vi "Publisher_SM.vi"() -> ()   [LabVIEW 2015]
uses:
  Data.ctl
  <vilib>/daq.io/MQTT LabVIEW Client/Controls/QoS.ctl
  <vilib>/daq.io/MQTT LabVIEW Client/Controls/Retain_Flag.ctl
  <vilib>/daq.io/MQTT LabVIEW Client/Controls/DUP_Flag.ctl
  <vilib>/daq.io/MQTT LabVIEW Client/Controls/Connection_Return_Codes.ctl
  Battery Controller.ctl
  States.ctl
  <vilib>/myRIO/Instrument Drivers/Onboard IO/DIO/typedefs/DIO Reference.ctl
  <vilib>/myRIO/Common/Instrument Driver Framework/Utilities/typedefs/myRIO Generic Hardware Reference.ctl
  <vilib>/myRIO/Common/Instrument Driver Framework/Utilities/typedefs/Hardware Version Enum.ctl
  <vilib>/myRIO/Common/Instrument Driver Framework/Utilities/typedefs/myRIO v1.0 Reference.ctl
  <vilib>/myRIO/Common/Instrument Driver Framework/Utilities/typedefs/Generic FPGA Reference.ctl
  <vilib>/myRIO/Common/Instrument Driver Framework/myRIO v1.0/DIO/typedefs/DIO Channels List.ctl
  <vilib>/myRIO/Common/Instrument Driver Framework/myRIO v1.0/DIO/typedefs/DIO Channels Enum.ctl
  <vilib>/userdefined/High Color/nirio_resource_hc.ctl
  <vilib>/myRIO/Common/Instrument Driver Framework/Utilities/vis/Is FPGA Ref Available.vi
  <vilib>/myRIO/Common/Instrument Driver Framework/myRIO v1.0/DIO/vis/myRIO v1.1 Open DIO.vi
  <vilib>/myRIO/Instrument Drivers/Onboard IO/DIO/vis/Read.vi
  <vilib>/myRIO/Instrument Drivers/Onboard IO/DIO/vis/Write.vi
  <vilib>/myRIO/Common/Instrument Driver Framework/Utilities/vis/Validate Channels.vi
  <vilib>/myRIO/Common/Instrument Driver Framework/myRIO v1.0/DIO/vis/myRIO v1.0 Reserve DIO.vi
  <vilib>/myRIO/Common/Instrument Driver Framework/myRIO v1.0/Resource Manager/vis/myRIO v1.0 Reserve Channel List.vi
  <vilib>/myRIO/Common/Instrument Driver Framework/myRIO v1.0/DIO/vis/myRIO v1.0 Build MUX Configuration DIO.vi
  <vilib>/myRIO/Common/Instrument Driver Framework/myRIO v1.0/Resource Manager/vis/myRIO v1.0 Reserve Channel.vi
  <vilib>/myRIO/Common/Instrument Driver Framework/myRIO v1.0/Resource Manager/vis/myRIO v1.0 Unreserve Channel.vi
  <vilib>/myRIO/Common/Instrument Driver Framework/myRIO v1.0/Resource Manager/vis/myRIO v1.0 Create Configuration List.vi
  <vilib>/myRIO/Common/Instrument Driver Framework/myRIO v1.0/Resource Manager/vis/myRIO v1.0 Build Mutex Name.vi
  <vilib>/Instr/_visa.llb/VISA Configure Serial Port (Instr).vi
  <vilib>/Utility/VariantDataType/GetNumericInfo.vi
  <vilib>/Utility/error.llb/Error Cluster From Error Code.vi
  <vilib>/myRIO/Common/Instrument Driver Framework/myRIO v1.0/myRIO v1.1 Open.vi
  <vilib>/myRIO/Common/Instrument Driver Framework/Utilities/vis/IO Manager.vi
  <vilib>/myRIO/Common/Instrument Driver Framework/Utilities/vis/Configuration Manager.vi
  <vilib>/myRIO/Common/Instrument Driver Framework/myRIO v1.0/Resource Manager/vis/myRIO v1.0 Configure IO.vi
  <vilib>/myRIO/Common/Instrument Driver Framework/myRIO v1.0/myRIO v1.0 Close.vi
  <vilib>/myRIO/Common/Instrument Driver Framework/myRIO v1.0/DIO/vis/myRIO v1.0 Read DIO.vi
  <vilib>/myRIO/Common/Instrument Driver Framework/myRIO v1.0/DIO/vis/myRIO v1.0 Write DIO.vi
  <vilib>/myRIO/Express VI/Onboard Devices/Button/Button Express VI.xnode
  <vilib>/myRIO/Instrument Drivers/Onboard IO/DIO/vis/myRIO DIO Open.xnode
  <vilib>/myRIO/Express VI/Onboard Devices/LED/LED Express VI.xnode
  <vilib>/daq.io/MQTT LabVIEW Client/MQTT_Functions.lvlib
  <vilib>/myRIO/Instrument Drivers/Onboard IO/DIO/DIO.lvlib
panel:
  in  "Battery Controls":T1={"Battery Serial Port"="ASRL2::INSTR", "Command to write"="RD_STAT>\r"}
  out "error out":errorcluster
  out "Session Status":string
  out "Published Data":string[][](array[string])
  in  "Stop Button":bool
  out "Connection Status":T2=enum."Connection refused: not authorized"
  in  "Connection Paramaters":T3={"VISA resource name"="ASRL1::INSTR", "myRIO AI Channel"=["C/AI0", "C/AI1"], "baud rate (9600)"=19200, "Write Command"="0R0!", "Client ID"="myRIO", "Topic"="All Weather Data", "Message ID"=10, "MQTT Broker"={"address (IP)"="52.38.228.154", "port"=1883}, "Publish Meta"={"QoS"=enum."At most once", "Retain"=FALSE, "DUP"=FALSE}, "TCP connection ID "=refnum, "Session Status"=""}
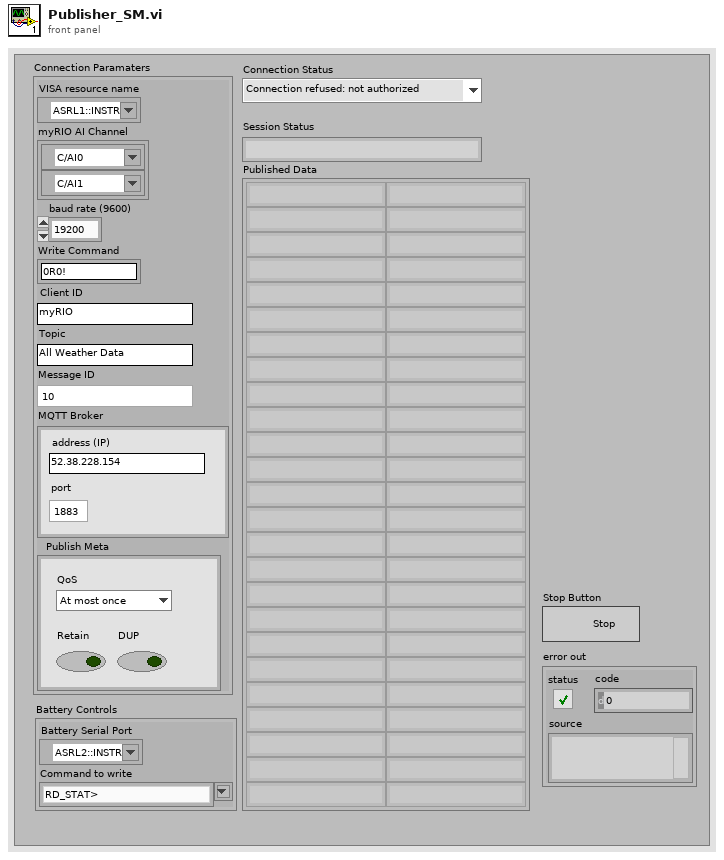
[diagram p1: front panel]
types:
  T1 = typedef "Battery Controller.ctl" = cluster{"Battery Serial Port":refnum<visa-resource-name>, "Command to write":string}
  T2 = typedef "MQTT_Functions.lvlib/Connection_Return_Codes.ctl" = enum16{"Connection accepted", "Connection refused: unacceptable protocol version", "Connection refused: identifier rejected", "Connection refused: Server unavailable", "Connection refused: bad user name or password", "Connection refused: not authorized"}
  T3 = typedef "Data.ctl" = cluster{"VISA resource name":refnum<visa-resource-name>, "myRIO AI Channel":tag[], "baud rate (9600)":u32, "Write Command":string, "Client ID":string, "Topic":string, "Message ID":u16, "MQTT Broker":cluster{"address (IP)":string, "port":u16}, "Publish Meta":cluster{"QoS":T4, "Retain":T5, "DUP":T6}, "TCP connection ID ":refnum<k5>, "Session Status":string}
  T4 = typedef "MQTT_Functions.lvlib/QoS.ctl" = enum8{"At most once", "At least once", "Exactly once", "Reserved"}
  T5 = typedef "MQTT_Functions.lvlib/Retain_Flag.ctl" = bool
  T6 = typedef "MQTT_Functions.lvlib/DUP_Flag.ctl" = bool
  T7 = typedef "States.ctl" = enum16{"Initialize", "TCP Connect", "Gather/Publish", "TCP Ping", "Exit/Disconnect"}
  T8 = typedef "DIO.lvlib/DIO Reference.ctl" = cluster{"myRIO Reference":T9, "DIO Channels List":T13}
  T9 = typedef "myRIO Generic Hardware Reference.ctl" = cluster{"myRIO Model":T10, "myRIO Hardware Reference":T11}
  T10 = typedef "Hardware Version Enum.ctl" = enum16{"Unknown", "myRIO-1900", "myRIO-1950", "roboRIO"}
  T11 = typedef "myRIO v1.0 Reference.ctl" = cluster{"Generic FPGA Reference":T12, "Allow multiple opens":bool}
  T12 = typedef "Generic FPGA Reference.ctl" = refnum<k20>
  T13 = typedef "DIO Channels List.ctl" = T14[]
  T14 = typedef "DIO Channels Enum.ctl" = enum16{"Not Connected", "C/DIO0", "C/DIO1", "C/DIO2", "C/DIO3", "C/DIO4", "C/DIO5", "C/DIO6", "C/DIO7", "A/DIO0", "A/DIO1", "A/DIO2", "A/DIO3", "A/DIO4", "A/DIO5", "A/DIO6", "A/DIO7", "A/DIO8", "A/DIO9", "A/DIO10", "A/DIO11", "A/DIO12", "A/DIO13", "A/DIO14", "A/DIO15", "B/DIO0", "B/DIO1", "B/DIO2", "B/DIO3", "B/DIO4", "B/DIO5", "B/DIO6", "B/DIO7", "B/DIO8", "B/DIO9", "B/DIO10", "B/DIO11", "B/DIO12", "B/DIO13", "B/DIO14", "B/DIO15", "LED0", "LED1", "LED2", "LED3", "Button0", "DIO/DIO0", "DIO/DIO1", "DIO/DIO2", "DIO/DIO3", "DIO/DIO4", "DIO/DIO5", "DIO/DIO6", "DIO/DIO7", "DIO/DIO8", "DIO/DIO9", "SPI/CS0", "SPI/CS1", "SPI/CS2", "SPI/CS3", "LED RADIO (Green)", "LED RADIO (Red)", "LED COMM (Green)", "LED COMM (Red)", "LED MODE (Green)", "LED MODE (Red)"}
  T15 = typedef "nirio_resource_hc.ctl" = tag
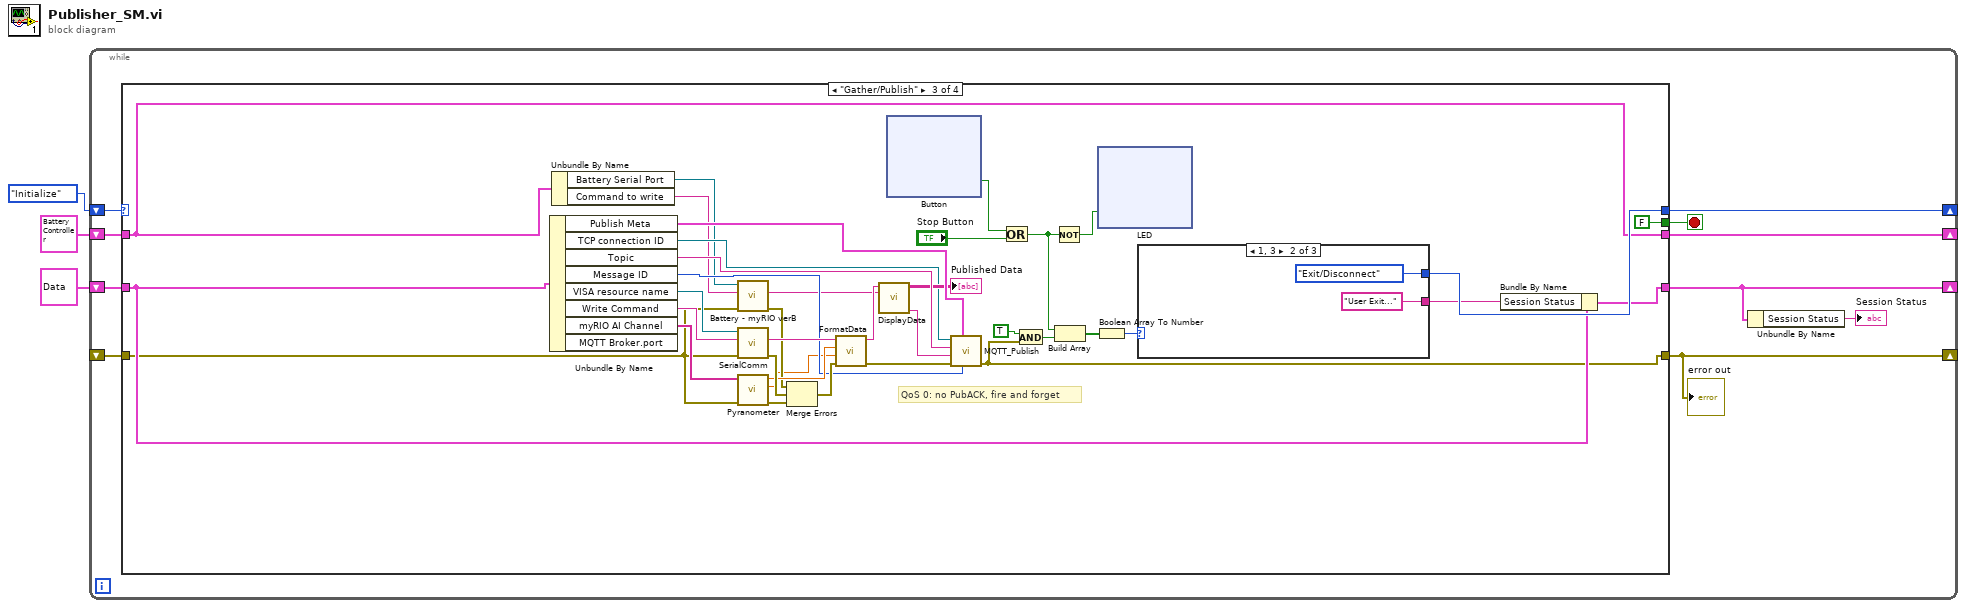
[diagram p0: block diagram]
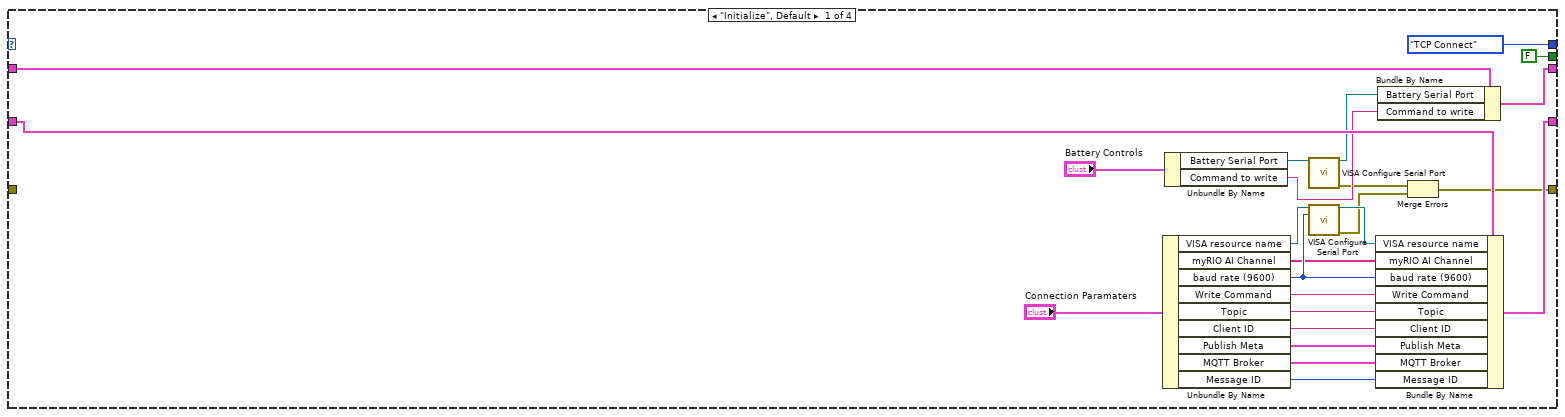
[diagram p2: hidden frame]
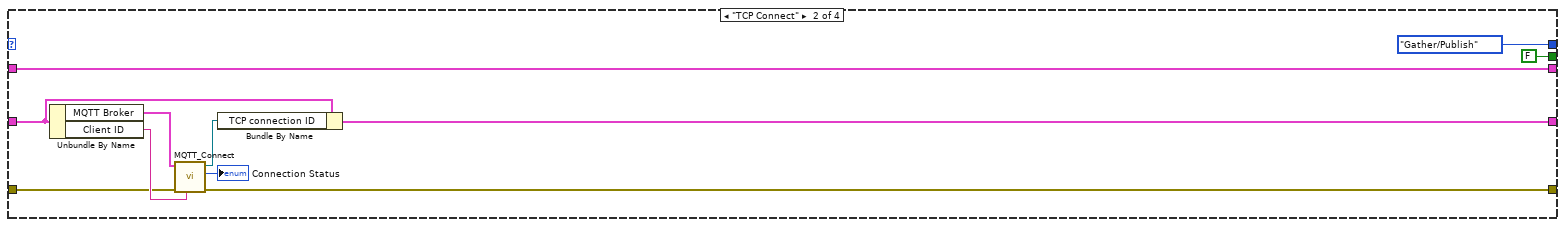
[diagram p3: hidden frame]
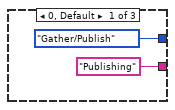
[diagram p4: hidden frame]
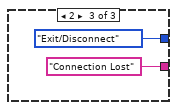
[diagram p5: hidden frame]
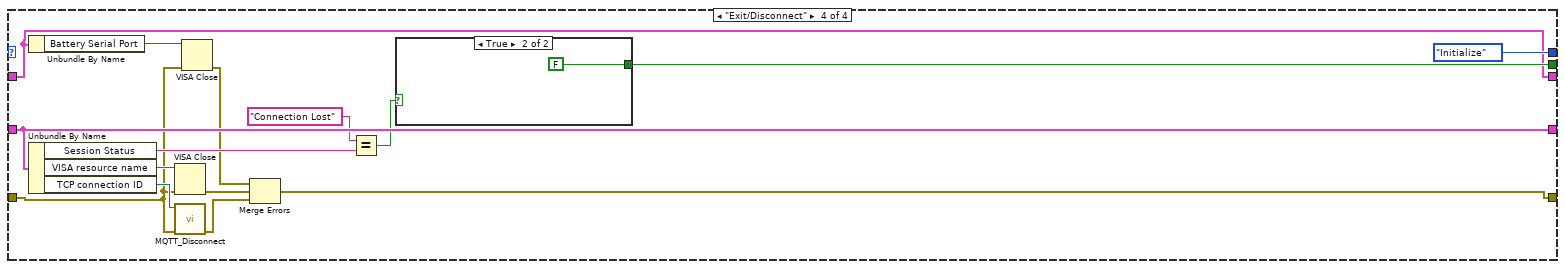
[diagram p6: hidden frame]
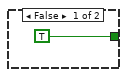
[diagram p7: hidden frame]
diagram:
  n1 = while {
    shift-right: [w13] -> _
    shift-left: States."Initialize" -> [w12]
    shift-right: [w8] -> _
    shift-left: T3 {"VISA resource name"="ASRL1::INSTR", "myRIO AI Channel"=["C/AI0"], "baud rate (9600)"=19200, "Write Command"="0R0!", "Client ID"="myRIO", "Topic"="data", "Message ID"=10, "MQTT Broker"={"address (IP)"="52.37.169.179", "port"=1883}, "Publish Meta"={"QoS"=enum."At most once", "Retain"=FALSE, "DUP"=FALSE}, "TCP connection ID "=refnum, "Session Status"=""} ("Cluster") -> [w11]
    shift-right: [w6] -> _
    shift-left: _ -> [w10]
    shift-right: [w4] -> _
    shift-left: T1 {"Battery Serial Port"="ASRL2::INSTR", "Command to write"="RD_STAT>\r"} ("Battery Controls") -> [w5]
    stop <- w9 stop-if-true
    n2 = case shown="\"Gather/Publish\"" w12 {
      tunnel: [States."TCP Connect" States."Gather/Publish" w74 States."Initialize"] -> w13
      tunnel: w11 -> [w36 w43 w69 w170]
      tunnel: [w24 w41 w68 w170] -> w8
      tunnel: [w14 w45 w67 w166] -> w6
      tunnel: w10 -> [_ w40 w52 w164]
      tunnel: [FALSE FALSE FALSE w171] -> w9
      tunnel: [w18 w38 w55 w162] -> w4
      tunnel: w5 -> [w20 w38 w55 w162]
      frame "Initialize", Default {
        n3 = Unbundle By Name("Connection Paramaters") -> ("VISA resource name"=w23:refnum<visa-resource-name>, "myRIO AI Channel"=w25:tag[], "baud rate (9600)"=w28:u32, "Write Command"=w29:string, "Topic"=w30:string, "Client ID"=w31:string, "Publish Meta"=w32:cluster{"QoS":T4, "Retain":T5, "DUP":T6}, "MQTT Broker"=w33:cluster{"address (IP)":string, "port":u16}, "Message ID"=w27:u16)
        n4 = Unbundle By Name("Battery Controls") -> ("Battery Serial Port"=w21:refnum<visa-resource-name>, "Command to write"=w17:string)
        n5 = call-poly "VISA Configure Serial Port"("VISA resource name"=w21) -> ("VISA resource name out"=w19:refnum<visa-resource-name>, "error out"=w15:errorcluster)  [unwired: 13 in]
        n6 = call-poly "VISA Configure Serial Port"("VISA resource name"=w23, "baud rate (9600)"=w28) -> ("VISA resource name out"=w35:refnum<visa-resource-name>, "error out"=w16:errorcluster)  [unwired: 12 in]
        n7 = Bundle By Name(cluster=w36, "VISA resource name"=w35, "myRIO AI Channel"=w25, "baud rate (9600)"=w28, "Write Command"=w29, "Topic"=w30, "Client ID"=w31, "Publish Meta"=w32, "MQTT Broker"=w33, "Message ID"=w27) -> (w24:T3)
        n8 = Bundle By Name(cluster=w20, "Battery Serial Port"=w19, "Command to write"=w17) -> (w18:T1)
        n9 = Merge Errors(w15, w16) -> (w14:errorcluster)
      }
      frame "TCP Connect" {
        n10 = Unbundle By Name(w43) -> ("MQTT Broker"=w47:cluster{"address (IP)":string, "port":u16}, "Client ID"=w46:string)
        n11 = call <vilib>:"MQTT_Connect.vi"("Client ID"=w46, "error in (no error)"=w40, "MQTT Broker"=w47) -> ("error out"=w45:errorcluster, "Connection Status"=→"Connection Status":T2, "connection ID out"=w42:refnum<k5>)  [unwired: 6 in]
        n12 = Bundle By Name(cluster=w43, "TCP connection ID"=w42) -> (w41:T3)
      }
      frame "Gather/Publish" {
        # "QoS 0: no PubACK, fire and forget"
        n13 = Unbundle By Name(w69) -> ("Publish Meta"=w77:cluster{"QoS":T4, "Retain":T5, "DUP":T6}, "TCP connection ID"=w61:refnum<k5>, "Topic"=w76:string, "Message ID"=w75:u16, "VISA resource name"=w82:refnum<visa-resource-name>, "Write Command"=w81:string, "myRIO AI Channel"=w72:tag[])  [unwired: 1 out]
        n14 = Unbundle By Name(w55) -> ("Battery Serial Port"=w54:refnum<visa-resource-name>, "Command to write"=w53:string)
        n15 = call "Battery - myRIO verB.vi"("Error input"=w52, "Command to write"=w53, "VISA resource name out"=w54) -> ("Error Out"=w51:errorcluster, "csv output"=w50:string)  [unwired: 5 in, 2 out]
        n16 = call "SerialComm.vi"("error in (no error)"=w52, "Write Command"=w81, "VISA Refnum in"=w82) -> ("error out"=w83:errorcluster, "Read Buffer"=w79:string)  [unwired: 6 in, 1 out]
        n17 = call "Pyranometer.vi"("error in (no error)"=w52, "Channel Names"=w72) -> ("error out"=w84:errorcluster, "Lower Irradiance"=w49:dbl, "Upper Irradiance"=w80:dbl)  [unwired: 7 in]
        n18 = Merge Errors(w51, w83, w84) -> (w85:errorcluster)
        n19 = call "FormatData.vi"("error in (no error)"=w85, "Lower Irradiance 2"=w49, "Upper Irradiance"=w80, "Read Buffer"=w79) -> ("error out"=w78:errorcluster, "CSV Output"=w71:string)  [unwired: 6 in]
        n20 = call "DisplayData.vi"("Battery Values"=w50, "Vaisala Input"=w71) -> ("CSV output"=w60:string, "Published Data"=→"Published Data":string[][])  [unwired: 8 in]
        n21 = xnode "Button"() -> ("Value"=w59:bool)  [unwired: 1 in, 1 out]
        n22 = call <vilib>:"MQTT_Publish.vi"("Message ID"=w75, "Publish Meta"=w77, "error in (no error)"=w78, "Message to be published"=w60, "Topic"=w76, "connection ID"=w61) -> ("error out"=w67:errorcluster)  [unwired: 4 in, 1 out]
        n23 = Or(x=w59, y="Stop Button") -> (x .or. y?=w57:bool)
        n24 = And(x=TRUE, y=w67) -> (x .and. y?=w62:bool)
        n25 = Not(x=w57) -> (.not. x?=w56:bool)
        n26 = Build Array(w57, w62) -> (w65:bool[])
        n27 = Boolean Array To Number(Boolean array=w65) -> (number=w64:u32)
        n28 = xnode "LED"("Status"=w56) -> ()  [unwired: 1 in, 1 out]
        n29 = case shown="1, 3" w64 {
          tunnel: [States."Gather/Publish" States."Exit/Disconnect" States."Exit/Disconnect"] -> w74
          tunnel: ["Publishing" ("Session Status") "User Exit..." ("Session Status") "Connection Lost" ("Session Status")] -> w63
          frame 0, Default {
          }
          frame 1, 3 {
          }
          frame 2 {
          }
        }
        n30 = Bundle By Name(cluster=w69, "Session Status"=w63) -> (w68:T3)
      }
      frame "Exit/Disconnect" {
        n31 = Unbundle By Name(w162) -> ("Battery Serial Port"=w165:refnum<visa-resource-name>)
        n32 = Unbundle By Name(w170) -> ("Session Status"=w167:string, "VISA resource name"=w176:refnum<visa-resource-name>, "TCP connection ID"=w173:refnum<k5>)
        n33 = VISA Close(VISA resource name=w176, error in (no error)=w164) -> (error out=w174:errorcluster)
        n34 = call <vilib>:"MQTT_Disconnect.vi"("error in (no error)"=w164, "connection ID"=w173) -> ("error out"=w175:errorcluster)  [unwired: 9 in]
        n35 = VISA Close(VISA resource name=w165, error in (no error)=w164) -> (error out=w163:errorcluster)
        n36 = Merge Errors(w163, w174, w175) -> (w166:errorcluster)
        n37 = Equal?(x="Connection Lost" ("Session Status"), y=w167) -> (x = y?=w168:bool)
        n38 = case shown="True" w168 {
          tunnel: [TRUE FALSE] -> w171
          frame False {
          }
          frame True {
          }
        }
      }
    }
    "error out" <- w6
    n39 = Unbundle By Name(w8) -> ("Session Status"=→"Session Status":string)
  }
